vi "Binary Data Log.vi"(9 "Error or Abort":bool, 11 "error in":errorcluster, 14 "Settings Cluster":T8={"Supply Voltage [Vdc]"=0.0, "Max Supply Current [Idc]"=0.0, "Settling Delay"=0.0, "Temp Criteria"=0.0, "Voltage Steps [Vrms]"=[], "User Notes"="", "Config Wave File Path"=path "", "Config Voltage [Vrms]"=0.0, "Channel Configuration List"={"Channel Configuration Cluster"={"Input"=enum."---", "Enable"=FALSE, "User Notes"="", "Voltage Range"=15.0, "Current Range"=2.5}, "Channel Configuration Cluster 2"={"Input"=enum."---", "Enable"=FALSE, "User Notes"="", "Voltage Range"=15.0, "Current Range"=2.5}, "Channel Configuration Cluster 3"={"Input"=enum."---", "Enable"=FALSE, "User Notes"="", "Voltage Range"=15.0, "Current Range"=2.5}, "Channel Configuration Cluster 4"={"Input"=enum."---", "Enable"=FALSE, "User Notes"="", "Voltage Range"=15.0, "Current Range"=2.5}, "Channel Configuration Cluster 5"={"Input"=enum."---", "Enable"=FALSE, "User Notes"="", "Voltage Range"=15.0, "Current Range"=2.5}, "Channel Configuration Cluster 6"={"Input"=enum."---", "Enable"=FALSE, "User Notes"="", "Voltage Range"=15.0, "Current Range"=2.5}, "Channel Configuration Cluster 7"={"Input"=enum."---", "Enable"=FALSE, "User Notes"="", "Voltage Range"=15.0, "Current Range"=2.5}, "Channel Configuration Cluster 8"={"Input"=enum."---", "Enable"=FALSE, "User Notes"="", "Voltage Range"=15.0, "Current Range"=2.5}, "Channel Configuration Cluster 9"={"Input"=enum."---", "Enable"=FALSE, "User Notes"="", "Voltage Range"=15.0, "Current Range"=2.5}, "Channel Configuration Cluster 10"={"Input"=enum."---", "Enable"=FALSE, "User Notes"="", "Voltage Range"=15.0, "Current Range"=2.5}, "Channel Configuration Cluster 11"={"Input"=enum."---", "Enable"=FALSE, "User Notes"="", "Voltage Range"=15.0, "Current Range"=2.5}, "Channel Configuration Cluster 12"={"Input"=enum."---", "Enable"=FALSE, "User Notes"="", "Voltage Range"=15.0, "Current Range"=2.5}, "Channel Configuration Cluster 13"={"Input"=enum."---", "Enable"=FALSE, "User Notes"="", "Voltage Range"=15.0, "Current Range"=2.5}, "Channel Configuration Cluster 14"={"Input"=enum."---", "Enable"=FALSE, "User Notes"="", "Voltage Range"=15.0, "Current Range"=2.5}, "Channel Configuration Cluster 15"={"Input"=enum."---", "Enable"=FALSE, "User Notes"="", "Voltage Range"=15.0, "Current Range"=2.5}, "Channel Configuration Cluster 16"={"Input"=enum."---", "Enable"=FALSE, "User Notes"="", "Voltage Range"=15.0, "Current Range"=2.5}, "Channel Configuration Cluster 17"={"Input"=enum."---", "Enable"=FALSE, "User Notes"="", "Voltage Range"=15.0, "Current Range"=2.5}}, "User Gains"={"Gain 1"=0.0, "Gain 2"=0.0, "Gain 3"=0.0, "Gain 4"=0.0, "Gain 5"=0.0, "Gain 6"=0.0}, "Gains"={"Gain 1"=0.0, "Gain 2"=0.0, "Gain 3"=0.0, "Gain 4"=0.0, "Gain 5"=0.0, "Gain 6"=0.0}, "Gain Array"={"Gain 1"=0.0, "Gain 2"=0.0, "Gain 3"=0.0, "Gain 4"=0.0, "Gain 5"=0.0, "Gain 6"=0.0, "Gain 7"=0.0, "Gain 8"=0.0, "Gain 9"=0.0, "Gain 10"=0.0, "Gain 11"=0.0, "Gain 12"=0.0, "Gain 13"=0.0, "Gain 14"=0.0, "Gain 15"=0.0, "Gain 16"=0.0, "Gain 17"=0.0}, "Wave File Path 1"=path "", "Wave File Path 2"=path "", "Wave File Path 3"=path "", "Wave File Path 4"=path "", "Range"=FALSE, "CF"=FALSE} {"Gain Array"."Gain 17" format="%.2f"; "Gain Array"."Gain 16" format="%.2f"; "Gain Array"."Gain 15" format="%.2f"; "Gain Array"."Gain 14" format="%.2f"; "Gain Array"."Gain 13" format="%.2f"; "Gain Array"."Gain 12" format="%.2f"; "Gain Array"."Gain 11" format="%.2f"; "Gain Array"."Gain 10" format="%.2f"; "Gain Array"."Gain 9" format="%.2f"; "Gain Array"."Gain 8" format="%.2f"; "Gain Array"."Gain 7" format="%.2f"; "Gain Array"."Gain 6" format="%.2f"; "Gain Array"."Gain 5" format="%.2f"; "Gain Array"."Gain 4" format="%.2f"; "Gain Array"."Gain 3" format="%.2f"; "Gain Array"."Gain 2" format="%.2f"; "Gain Array"."Gain 1" format="%.2f"; "Gains"."Gain 6" format="%.2f"; "Gains"."Gain 5" format="%.2f"; "Gains"."Gain 4" format="%.2f"; "Gains"."Gain 3" format="%.2f"; "Gains"."Gain 2" format="%.2f"; "Gains"."Gain 1" format="%.2f"; "User Gains"."Gain 6" format="%.2f"; "User Gains"."Gain 5" format="%.2f"; "User Gains"."Gain 4" format="%.2f"; "User Gains"."Gain 3" format="%.2f"; "User Gains"."Gain 2" format="%.2f"; "User Gains"."Gain 1" format="%.2f"; "Channel Configuration List"."Channel Configuration Cluster 17"."Current Range" items=["1 <500m>"=0.5, "2 <1>"=1.0, "5 <2.5>"=2.5, "10 <5>"=5.0, "20 <10>"=10.0, "50 <25>"=25.0]; "Channel Configuration List"."Channel Configuration Cluster 17"."Voltage Range" items=["1.5 <0.75>"=0.75, "3 <1.5>"=1.5, "6 <3>"=3.0, "10 <5>"=5.0, "15 <7.5>"=7.5, "30 <15>"=15.0, "60 <30>"=30.0, "100 <50>"=50.0, "150 <75>"=75.0, "300 <150>"=150.0, "600 <300>"=300.0, "1000 <500>"=500.0]; "Channel Configuration List"."Channel Configuration Cluster 16"."Current Range" items=["1 <500m>"=0.5, "2 <1>"=1.0, "5 <2.5>"=2.5, "10 <5>"=5.0, "20 <10>"=10.0, "50 <25>"=25.0]; "Channel Configuration List"."Channel Configuration Cluster 16"."Voltage Range" items=["1.5 <0.75>"=0.75, "3 <1.5>"=1.5, "6 <3>"=3.0, "10 <5>"=5.0, "15 <7.5>"=7.5, "30 <15>"=15.0, "60 <30>"=30.0, "100 <50>"=50.0, "150 <75>"=75.0, "300 <150>"=150.0, "600 <300>"=300.0, "1000 <500>"=500.0]; "Channel Configuration List"."Channel Configuration Cluster 15"."Current Range" items=["1 <500m>"=0.5, "2 <1>"=1.0, "5 <2.5>"=2.5, "10 <5>"=5.0, "20 <10>"=10.0, "50 <25>"=25.0]; "Channel Configuration List"."Channel Configuration Cluster 15"."Voltage Range" items=["1.5 <0.75>"=0.75, "3 <1.5>"=1.5, "6 <3>"=3.0, "10 <5>"=5.0, "15 <7.5>"=7.5, "30 <15>"=15.0, "60 <30>"=30.0, "100 <50>"=50.0, "150 <75>"=75.0, "300 <150>"=150.0, "600 <300>"=300.0, "1000 <500>"=500.0]; "Channel Configuration List"."Channel Configuration Cluster 14"."Current Range" items=["1 <500m>"=0.5, "2 <1>"=1.0, "5 <2.5>"=2.5, "10 <5>"=5.0, "20 <10>"=10.0, "50 <25>"=25.0]; "Channel Configuration List"."Channel Configuration Cluster 14"."Voltage Range" items=["1.5 <0.75>"=0.75, "3 <1.5>"=1.5, "6 <3>"=3.0, "10 <5>"=5.0, "15 <7.5>"=7.5, "30 <15>"=15.0, "60 <30>"=30.0, "100 <50>"=50.0, "150 <75>"=75.0, "300 <150>"=150.0, "600 <300>"=300.0, "1000 <500>"=500.0]; "Channel Configuration List"."Channel Configuration Cluster 13"."Current Range" items=["1 <500m>"=0.5, "2 <1>"=1.0, "5 <2.5>"=2.5, "10 <5>"=5.0, "20 <10>"=10.0, "50 <25>"=25.0]; "Channel Configuration List"."Channel Configuration Cluster 13"."Voltage Range" items=["1.5 <0.75>"=0.75, "3 <1.5>"=1.5, "6 <3>"=3.0, "10 <5>"=5.0, "15 <7.5>"=7.5, "30 <15>"=15.0, "60 <30>"=30.0, "100 <50>"=50.0, "150 <75>"=75.0, "300 <150>"=150.0, "600 <300>"=300.0, "1000 <500>"=500.0]; "Channel Configuration List"."Channel Configuration Cluster 12"."Current Range" items=["1 <500m>"=0.5, "2 <1>"=1.0, "5 <2.5>"=2.5, "10 <5>"=5.0, "20 <10>"=10.0, "50 <25>"=25.0]; "Channel Configuration List"."Channel Configuration Cluster 12"."Voltage Range" items=["1.5 <0.75>"=0.75, "3 <1.5>"=1.5, "6 <3>"=3.0, "10 <5>"=5.0, "15 <7.5>"=7.5, "30 <15>"=15.0, "60 <30>"=30.0, "100 <50>"=50.0, "150 <75>"=75.0, "300 <150>"=150.0, "600 <300>"=300.0, "1000 <500>"=500.0]; "Channel Configuration List"."Channel Configuration Cluster 11"."Current Range" items=["1 <500m>"=0.5, "2 <1>"=1.0, "5 <2.5>"=2.5, "10 <5>"=5.0, "20 <10>"=10.0, "50 <25>"=25.0]; "Channel Configuration List"."Channel Configuration Cluster 11"."Voltage Range" items=["1.5 <0.75>"=0.75, "3 <1.5>"=1.5, "6 <3>"=3.0, "10 <5>"=5.0, "15 <7.5>"=7.5, "30 <15>"=15.0, "60 <30>"=30.0, "100 <50>"=50.0, "150 <75>"=75.0, "300 <150>"=150.0, "600 <300>"=300.0, "1000 <500>"=500.0]; "Channel Configuration List"."Channel Configuration Cluster 10"."Current Range" items=["1 <500m>"=0.5, "2 <1>"=1.0, "5 <2.5>"=2.5, "10 <5>"=5.0, "20 <10>"=10.0, "50 <25>"=25.0]; "Channel Configuration List"."Channel Configuration Cluster 10"."Voltage Range" items=["1.5 <0.75>"=0.75, "3 <1.5>"=1.5, "6 <3>"=3.0, "10 <5>"=5.0, "15 <7.5>"=7.5, "30 <15>"=15.0, "60 <30>"=30.0, "100 <50>"=50.0, "150 <75>"=75.0, "300 <150>"=150.0, "600 <300>"=300.0, "1000 <500>"=500.0]; "Channel Configuration List"."Channel Configuration Cluster 9"."Voltage Range" items=["1.5 <0.75>"=0.75, "3 <1.5>"=1.5, "6 <3>"=3.0, "10 <5>"=5.0, "15 <7.5>"=7.5, "30 <15>"=15.0, "60 <30>"=30.0, "100 <50>"=50.0, "150 <75>"=75.0, "300 <150>"=150.0, "600 <300>"=300.0, "1000 <500>"=500.0]; "Channel Configuration List"."Channel Configuration Cluster 9"."Current Range" items=["10m <5m>"=0.005, "20m <10m>"=0.01, "50m <25m>"=0.025, "100m <50m>"=0.05, "200m <100m>"=0.1, "500m <250m>"=0.25, "1 <500m>"=0.5, "2 <1>"=1.0, "5 <2.5>"=2.5]; "Channel Configuration List"."Channel Configuration Cluster 8"."Voltage Range" items=["1.5 <0.75>"=0.75, "3 <1.5>"=1.5, "6 <3>"=3.0, "10 <5>"=5.0, "15 <7.5>"=7.5, "30 <15>"=15.0, "60 <30>"=30.0, "100 <50>"=50.0, "150 <75>"=75.0, "300 <150>"=150.0, "600 <300>"=300.0, "1000 <500>"=500.0]; "Channel Configuration List"."Channel Configuration Cluster 8"."Current Range" items=["10m <5m>"=0.005, "20m <10m>"=0.01, "50m <25m>"=0.025, "100m <50m>"=0.05, "200m <100m>"=0.1, "500m <250m>"=0.25, "1 <500m>"=0.5, "2 <1>"=1.0, "5 <2.5>"=2.5]; "Channel Configuration List"."Channel Configuration Cluster 7"."Voltage Range" items=["1.5 <0.75>"=0.75, "3 <1.5>"=1.5, "6 <3>"=3.0, "10 <5>"=5.0, "15 <7.5>"=7.5, "30 <15>"=15.0, "60 <30>"=30.0, "100 <50>"=50.0, "150 <75>"=75.0, "300 <150>"=150.0, "600 <300>"=300.0, "1000 <500>"=500.0]; "Channel Configuration List"."Channel Configuration Cluster 7"."Current Range" items=["10m <5m>"=0.005, "20m <10m>"=0.01, "50m <25m>"=0.025, "100m <50m>"=0.05, "200m <100m>"=0.1, "500m <250m>"=0.25, "1 <500m>"=0.5, "2 <1>"=1.0, "5 <2.5>"=2.5]; "Channel Configuration List"."Channel Configuration Cluster 6"."Voltage Range" items=["1.5 <0.75>"=0.75, "3 <1.5>"=1.5, "6 <3>"=3.0, "10 <5>"=5.0, "15 <7.5>"=7.5, "30 <15>"=15.0, "60 <30>"=30.0, "100 <50>"=50.0, "150 <75>"=75.0, "300 <150>"=150.0, "600 <300>"=300.0, "1000 <500>"=500.0]; "Channel Configuration List"."Channel Configuration Cluster 6"."Current Range" items=["10m <5m>"=0.005, "20m <10m>"=0.01, "50m <25m>"=0.025, "100m <50m>"=0.05, "200m <100m>"=0.1, "500m <250m>"=0.25, "1 <500m>"=0.5, "2 <1>"=1.0, "5 <2.5>"=2.5]; "Channel Configuration List"."Channel Configuration Cluster 5"."Voltage Range" items=["1.5 <0.75>"=0.75, "3 <1.5>"=1.5, "6 <3>"=3.0, "10 <5>"=5.0, "15 <7.5>"=7.5, "30 <15>"=15.0, "60 <30>"=30.0, "100 <50>"=50.0, "150 <75>"=75.0, "300 <150>"=150.0, "600 <300>"=300.0, "1000 <500>"=500.0]; "Channel Configuration List"."Channel Configuration Cluster 5"."Current Range" items=["10m <5m>"=0.005, "20m <10m>"=0.01, "50m <25m>"=0.025, "100m <50m>"=0.05, "200m <100m>"=0.1, "500m <250m>"=0.25, "1 <500m>"=0.5, "2 <1>"=1.0, "5 <2.5>"=2.5]; "Channel Configuration List"."Channel Configuration Cluster 4"."Voltage Range" items=["1.5 <0.75>"=0.75, "3 <1.5>"=1.5, "6 <3>"=3.0, "10 <5>"=5.0, "15 <7.5>"=7.5, "30 <15>"=15.0, "60 <30>"=30.0, "100 <50>"=50.0, "150 <75>"=75.0, "300 <150>"=150.0, "600 <300>"=300.0, "1000 <500>"=500.0]; "Channel Configuration List"."Channel Configuration Cluster 4"."Current Range" items=["10m <5m>"=0.005, "20m <10m>"=0.01, "50m <25m>"=0.025, "100m <50m>"=0.05, "200m <100m>"=0.1, "500m <250m>"=0.25, "1 <500m>"=0.5, "2 <1>"=1.0, "5 <2.5>"=2.5]; "Channel Configuration List"."Channel Configuration Cluster 3"."Voltage Range" items=["1.5 <0.75>"=0.75, "3 <1.5>"=1.5, "6 <3>"=3.0, "10 <5>"=5.0, "15 <7.5>"=7.5, "30 <15>"=15.0, "60 <30>"=30.0, "100 <50>"=50.0, "150 <75>"=75.0, "300 <150>"=150.0, "600 <300>"=300.0, "1000 <500>"=500.0]; "Channel Configuration List"."Channel Configuration Cluster 3"."Current Range" items=["10m <5m>"=0.005, "20m <10m>"=0.01, "50m <25m>"=0.025, "100m <50m>"=0.05, "200m <100m>"=0.1, "500m <250m>"=0.25, "1 <500m>"=0.5, "2 <1>"=1.0, "5 <2.5>"=2.5]; "Channel Configuration List"."Channel Configuration Cluster 2"."Voltage Range" items=["1.5 <0.75>"=0.75, "3 <1.5>"=1.5, "6 <3>"=3.0, "10 <5>"=5.0, "15 <7.5>"=7.5, "30 <15>"=15.0, "60 <30>"=30.0, "100 <50>"=50.0, "150 <75>"=75.0, "300 <150>"=150.0, "600 <300>"=300.0, "1000 <500>"=500.0]; "Channel Configuration List"."Channel Configuration Cluster 2"."Current Range" items=["10m <5m>"=0.005, "20m <10m>"=0.01, "50m <25m>"=0.025, "100m <50m>"=0.05, "200m <100m>"=0.1, "500m <250m>"=0.25, "1 <500m>"=0.5, "2 <1>"=1.0, "5 <2.5>"=2.5]; "Channel Configuration List"."Channel Configuration Cluster"."Voltage Range" items=["1.5 <0.75>"=0.75, "3 <1.5>"=1.5, "6 <3>"=3.0, "10 <5>"=5.0, "15 <7.5>"=7.5, "30 <15>"=15.0, "60 <30>"=30.0, "100 <50>"=50.0, "150 <75>"=75.0, "300 <150>"=150.0, "600 <300>"=300.0, "1000 <500>"=500.0]; "Channel Configuration List"."Channel Configuration Cluster"."Current Range" items=["10m <5m>"=0.005, "20m <10m>"=0.01, "50m <25m>"=0.025, "100m <50m>"=0.05, "200m <100m>"=0.1, "500m <250m>"=0.25, "1 <500m>"=0.5, "2 <1>"=1.0, "5 <2.5>"=2.5]; "Settling Delay" min=0.0 format="%<%H:%M:%S>t"}) -> (15 "error out":errorcluster)   [LabVIEW 2015]
uses:
  Controls/Settings Control.ctl
  Controls/Channel Configuration Cluster.ctl
  Controls/Channel Configuration List.ctl
  Controls/Gain Averages.ctl
  Controls/Gain Array.ctl
  Controls/Datalog Bundle Control.ctl
  Controls/DSA Readings.ctl
  Controls/DSA Measurements.ctl
  Controls/DSA Functions.ctl
  Controls/WT1800 Readings.ctl
  Controls/WT1800 Measurements.ctl
  Controls/WT1800 Functions.ctl
  Controls/Channel Configuration Cluster High Current.ctl
panel:
  in  "Datalog Cluster Array":T1[](array[typedef])=[{"Heat"=0.0, "WT1800 Functions"=[], "WT1800 Averages"=[], "WT1800 Measurements"=[], "DSA Functions"=[], "DSA Averages"=[], "DSA Measurements"=[], "Initial Time Stamp"=timestamp(0 s since 1904-01-01), "Final Time Stamp"=timestamp(0 s since 1904-01-01), "Temperature Data"=[]}] {"WT1800 Averages"."Vrms" format="%.3f"; "WT1800 Averages"."Irms" format="%.3f"; "WT1800 Averages"."Power" format="%.3f"; "WT1800 Averages"."Vpkpk" format="%.3f"; "WT1800 Averages"."Ipkpk" format="%.3f"; "WT1800 Measurements"."Vrms" format="%.3f"; "WT1800 Measurements"."Irms" format="%.3f"; "WT1800 Measurements"."Power" format="%.3f"; "WT1800 Measurements"."Vpkpk" format="%.3f"; "WT1800 Measurements"."Ipkpk" format="%.3f"; "DSA Averages"."Vrms" format="%.3f"; "DSA Averages"."Vdc" format="%.3f"; "DSA Averages"."Vpk+" format="%.3f"; "DSA Averages"."Vpk-" format="%.3f"; "DSA Averages"."Vpkpk" format="%.3f"; "DSA Measurements"."Vrms" format="%.3f"; "DSA Measurements"."Vdc" format="%.3f"; "DSA Measurements"."Vpk+" format="%.3f"; "DSA Measurements"."Vpk-" format="%.3f"; "DSA Measurements"."Vpkpk" format="%.3f"}
  in  "Template Path":path
  in  "Z_JPEG_path":path
  in  "EQ_JPEG_path":path
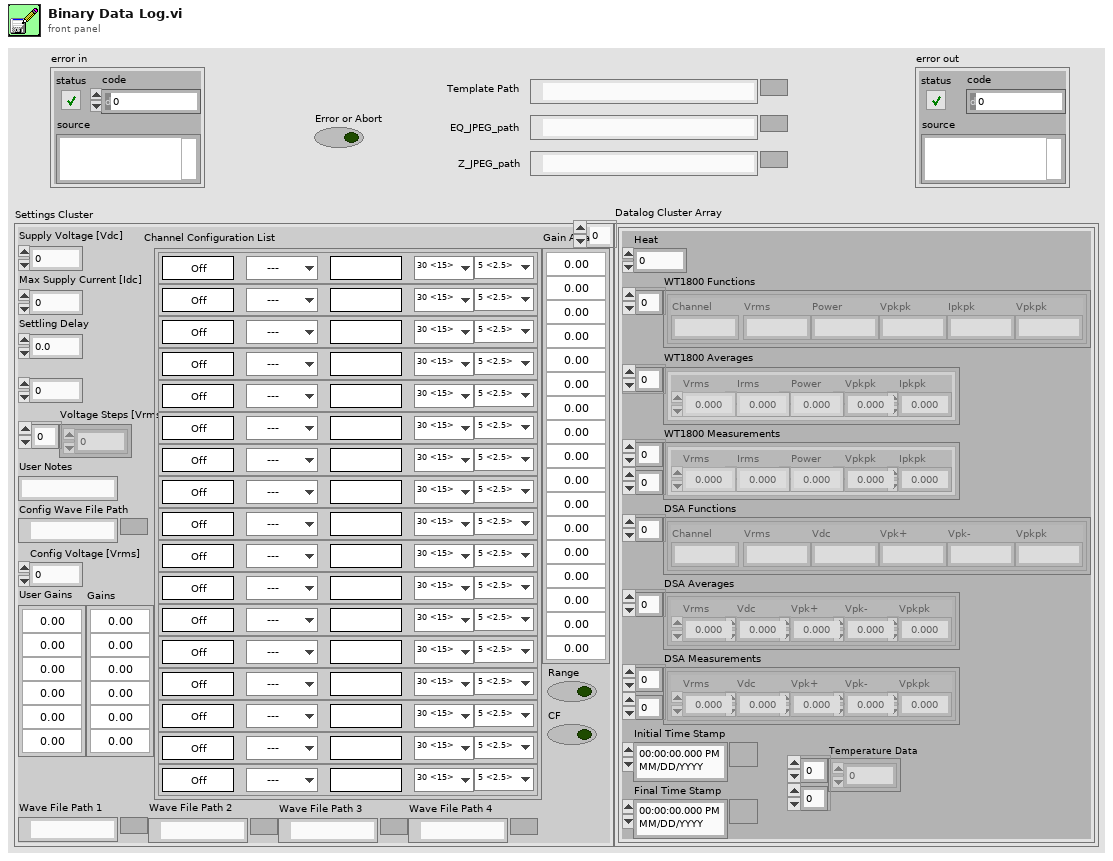
[diagram p1: front panel]
types:
  T1 = typedef "Datalog Bundle Control.ctl" = cluster{"Heat":dbl, "WT1800 Functions":T2, "WT1800 Averages":T3, "WT1800 Measurements":T4[][], "DSA Functions":T5, "DSA Averages":T6, "DSA Measurements":T7[][], "Initial Time Stamp":timestamp, "Final Time Stamp":timestamp, "Temperature Data":dbl[][]}
  T2 = typedef "WT1800 Functions.ctl" = cluster{"Channel":string, "Vrms":string, "Power":string, "Vpkpk":string, "Ipkpk":string, "Vpkpk":string}[]
  T3 = typedef "WT1800 Measurements.ctl" = T4[]
  T4 = typedef "WT1800 Readings.ctl" = cluster{"Vrms":dbl, "Irms":dbl, "Power":dbl, "Vpkpk":dbl, "Ipkpk":dbl}
  T5 = typedef "DSA Functions.ctl" = cluster{"Channel":string, "Vrms":string, "Vdc":string, "Vpk+":string, "Vpk-":string, "Vpkpk":string}[]
  T6 = typedef "DSA Measurements.ctl" = T7[]
  T7 = typedef "DSA Readings.ctl" = cluster{"Vrms":dbl, "Vdc":dbl, "Vpk+":dbl, "Vpk-":dbl, "Vpkpk":dbl}
  T8 = typedef "Settings Control.ctl" = cluster{"Supply Voltage [Vdc]":dbl, "Max Supply Current [Idc]":dbl, "Settling Delay":dbl, "Temp Criteria":dbl, "Voltage Steps [Vrms]":dbl[], "User Notes":string, "Config Wave File Path":path, "Config Voltage [Vrms]":dbl, "Channel Configuration List":T9, "User Gains":T12, "Gains":T12, "Gain Array":T13, "Wave File Path 1":path, "Wave File Path 2":path, "Wave File Path 3":path, "Wave File Path 4":path, "Range":bool, "CF":bool}
  T9 = typedef "Channel Configuration List.ctl" = cluster{"Channel Configuration Cluster":T10, "Channel Configuration Cluster 2":T10, "Channel Configuration Cluster 3":T10, "Channel Configuration Cluster 4":T10, "Channel Configuration Cluster 5":T10, "Channel Configuration Cluster 6":T10, "Channel Configuration Cluster 7":T10, "Channel Configuration Cluster 8":T10, "Channel Configuration Cluster 9":T10, "Channel Configuration Cluster 10":T11, "Channel Configuration Cluster 11":T11, "Channel Configuration Cluster 12":T11, "Channel Configuration Cluster 13":T11, "Channel Configuration Cluster 14":T11, "Channel Configuration Cluster 15":T11, "Channel Configuration Cluster 16":T11, "Channel Configuration Cluster 17":T11}
  T10 = typedef "Channel Configuration Cluster.ctl" = cluster{"Input":enum16{"---", "1", "1 AVG", "2", "2 AVG", "3", "3 AVG", "4", "4 AVG"}, "Enable":bool, "User Notes":string, "Voltage Range":dbl, "Current Range":dbl}
  T11 = typedef "Channel Configuration Cluster High Current.ctl" = cluster{"Input":enum16{"---", "1", "1 AVG", "2", "2 AVG", "3", "3 AVG", "4", "4 AVG"}, "Enable":bool, "User Notes":string, "Voltage Range":dbl, "Current Range":dbl}
  T12 = typedef "Gain Averages.ctl" = cluster{"Gain 1":dbl, "Gain 2":dbl, "Gain 3":dbl, "Gain 4":dbl, "Gain 5":dbl, "Gain 6":dbl}
  T13 = typedef "Gain Array.ctl" = cluster{"Gain 1":dbl, "Gain 2":dbl, "Gain 3":dbl, "Gain 4":dbl, "Gain 5":dbl, "Gain 6":dbl, "Gain 7":dbl, "Gain 8":dbl, "Gain 9":dbl, "Gain 10":dbl, "Gain 11":dbl, "Gain 12":dbl, "Gain 13":dbl, "Gain 14":dbl, "Gain 15":dbl, "Gain 16":dbl, "Gain 17":dbl}
  T14 = enum16{"open", "replace", "create", "open or create", "replace or create", "replace or create with confirmation"}
  T15 = cluster{"Template Path":path, "EQ_JPEG_path":path, "Z_JPEG_path":path, "Settings Cluster":T8, dbl[], "WT1800 Functions":cluster{"Channel":string, "Vrms":string, "Power":string, "Vpkpk":string, "Ipkpk":string, "Vpkpk":string}[][], "WT1800 Averages":T4[][], "WT1800 Measurements":T4[][][], "DSA Functions":cluster{"Channel":string, "Vrms":string, "Vdc":string, "Vpk+":string, "Vpk-":string, "Vpkpk":string}[][], "DSA Averages":T7[][], "DSA Measurements":T7[][][], timestamp[], timestamp[]}
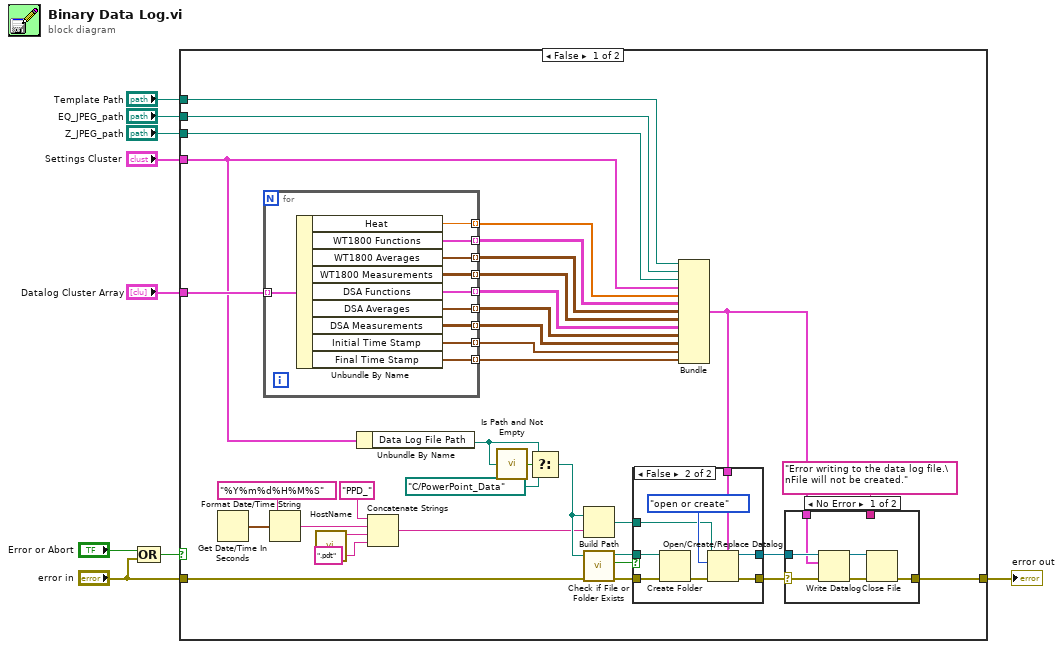
[diagram p0: block diagram]
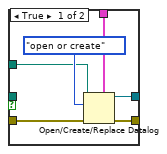
[diagram p2: hidden frame]
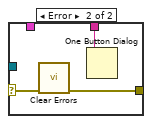
[diagram p3: hidden frame]
diagram:
  n1 = Compound Arithmetic op=OR("Error or Abort", "error in") -> (w5:bool)
  n2 = case shown="False" w5 {
    tunnel: [w44 w78] -> w9
    tunnel: "error in" -> [w38 w78]
    tunnel: "Settings Cluster" -> [w11 _]
    tunnel: "EQ_JPEG_path" -> [w24 _]
    tunnel: "Template Path" -> [w23 _]
    tunnel: "Z_JPEG_path" -> [w22 _]
    tunnel: "Datalog Cluster Array" -> [w21 _]
    frame False {
      n3 = Get Date/Time In Seconds() -> (seconds since 1Jan1904=w10:timestamp)
      n4 = for {
        tunnel: w21 -> [w54] mode=indexing
        tunnel: [w53] -> w20 mode=indexing
        tunnel: [w52] -> w19 mode=indexing
        tunnel: [w51] -> w18 mode=indexing
        tunnel: [w50] -> w17 mode=indexing
        tunnel: [w49] -> w16 mode=indexing
        tunnel: [w48] -> w15 mode=indexing
        tunnel: [w47] -> w14 mode=indexing
        tunnel: [w46] -> w13 mode=indexing
        tunnel: [w45] -> w12 mode=indexing
        n5 = Unbundle By Name(w54) -> ("Heat"=w53:dbl, "WT1800 Functions"=w52:T2, "WT1800 Averages"=w51:T3, "WT1800 Measurements"=w50:T4[][], "DSA Functions"=w49:T5, "DSA Averages"=w48:T6, "DSA Measurements"=w47:T7[][], "Initial Time Stamp"=w46:timestamp, "Final Time Stamp"=w45:timestamp)
      }
      n6 = Format Date/Time String(time format string (%c)="%Y%m%d%H%M%S", seconds (now)=w10) -> (date/time string=w29:string)  [unwired: 1 in]
      n7 = call "HostName.vi"() -> ("String/Binary data"=w30:string)  [unwired: 10 in, 1 out]
      n8 = Unbundle By Name(w11) -> ("Data Log File Path"=w34:path)
      n9 = Concatenate Strings("PPD_" ("name or relative path"), w29, w30, ".pdt" ("Substring")) -> (w26:string)
      n10 = call <vilib>:"Is Path and Not Empty.vi"("path"=w34) -> ("Is Path and Not Empty?"=w42:bool)  [unwired: 4 in]
      n11 = Select(t=w34, s=w42, f=path "C:/PowerPoint_Data") -> (s? t:f=w32:path)
      n12 = Build Path(base path=w32, name or relative path=w26) -> (appended path=w33:path)
      n13 = call <vilib>:"Check if File or Folder Exists.vi"("error in (no error)"=w38, "path"=w32) -> ("error out"=w37:errorcluster, "file or folder exists?"=w35:bool, "dup path"=w36:path)  [unwired: 7 in]
      n14 = Bundle("Template Path"=w23, "EQ_JPEG_path"=w24, "Z_JPEG_path"=w22, "Settings Cluster"=w11, w20, "WT1800 Functions"=w19, "WT1800 Averages"=w18, "WT1800 Measurements"=w17, "DSA Functions"=w16, "DSA Averages"=w15, "DSA Measurements"=w14, w13, w12) -> (w25:T15)  [unwired: 1 in]
      n15 = case shown="False" w35 {
        tunnel: w25 -> [w60 w68]
        tunnel: [w58 w66] -> w43
        tunnel: [w57 w65] -> w40
        tunnel: w37 -> [w56 w64]
        tunnel: w36 -> [_ w62]
        tunnel: w33 -> [w55 w61]
        frame True {
          n16 = Open/Create/Replace Datalog(5:w60, 8:w56, 10:T14."open or create" ("operation (0:open)"), 11:w55) -> (0:w57:errorcluster, 3:w58:refnum<k1>)  [unwired: 3 out]
        }
        frame False {
          n17 = Create Folder(path (use dialog)=w62, error in=w64) -> (error out=w63:errorcluster)  [unwired: 1 in, 2 out]
          n18 = Open/Create/Replace Datalog(5:w68, 8:w63, 10:T14."open or create" ("operation (0:open)"), 11:w61) -> (0:w65:errorcluster, 3:w66:refnum<k1>)  [unwired: 3 out]
        }
      }
      n19 = case shown="No Error" w40 {
        selector: w40 -> [w69 w76]
        tunnel: [w72 w75] -> w44
        tunnel: w43 -> [w71 _]
        tunnel: w25 -> [w70 _]
        tunnel: "Error writing to the data log file.\nFile will not be created." ("message") -> [_ w77]
        frame No Error {
          n20 = Write Datalog(4:w69, 6:w70, 7:w71) -> (0:w74:errorcluster, 3:w73:refnum<k1>)
          n21 = Close File(refnum=w73, error in=w74) -> (error out=w72:errorcluster)  [unwired: 1 out]
        }
        frame Error {
          n22 = call <vilib>:"Clear Errors.vi"("error in (no error)"=w76) -> ("error out"=w75:errorcluster)  [unwired: 5 in, 1 out]
          n23 = One Button Dialog(message=w77) -> ()  [unwired: 1 in, 1 out]
        }
      }
    }
    frame True {
    }
  }
  "error out" <- w9
